vi "LV MySQL Example.vi"() -> ()   [LabVIEW 2010]
uses:
  typedefs/mysql_authentication.ctl
panel:
  in  "Port":u16=3306
  in  "IP Address":string="localhost"
  in  "Authentication":T1={"User"="root", "Password"="fabregas", "Database"="netlab"}
  out "data":string[][](array[string])
  out "error out":errorcluster={"status"=TRUE, "code"=5000, "source"="1146 | #42S02Table 'netlab.data' doesn't exist"}
  in  "Query":string="SELECT * FROM data"
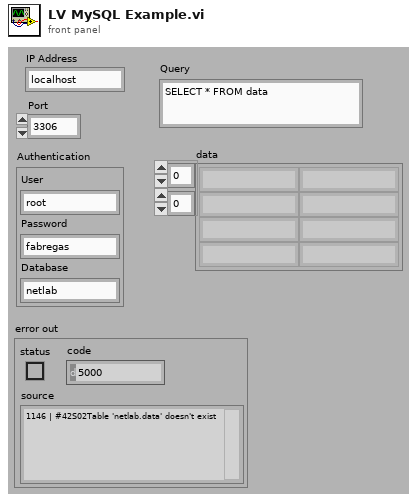
[diagram p1: front panel]
types:
  T1 = typedef "mysql_authentication.ctl" = cluster{"User":string, "Password":string, "Database":string}
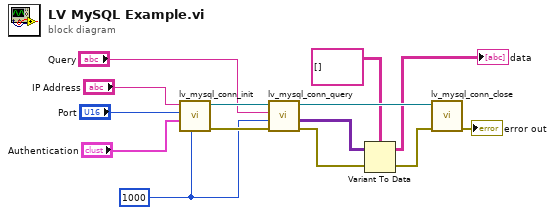
[diagram p0: block diagram]
diagram:
  w8 = 1000 ("timeout ms (60000)")
  n1 = call "lv_mysql_conn_init.vi"("timeout ms (5000)"=w8, "Authentication"="Authentication", "Port"="Port", "IP Address"="IP Address") -> ("error out"=w11:errorcluster, "connection ID out"=w10:refnum<k5>)  [unwired: 6 in]
  n2 = call "lv_mysql_conn_query.vi"("error in (no error)"=w11, "timeout ms (5000)"=w8, "Query"="Query", "connection ID"=w10) -> ("error out"=w2:errorcluster, "Return Data"=w5:variant[][], "connection ID out"=w9:refnum<k5>)  [unwired: 4 in, 1 out]
  n3 = Variant To Data(error in=w2, Variant=w5, type=string[][] []) -> (error out=w1:errorcluster, data=→"data":string[][])
  n4 = call "lv_mysql_conn_close.vi"("error in (no error)"=w1, "connection ID"=w9) -> ("error out"=→"error out":errorcluster)  [unwired: 9 in]
